vi "DrawPathAndRobotOnThatPath.vi"(6 "CenterOfRotYOffset (px)":dbl=20.0, 7 "PathMode":enum16{"Left", "Right", "Center"}(ring)=enum."Center", 8 "RobotLength (px)":dbl=40.0, 9 "RobotWidth (px)":dbl=30.0, 10 "Path (px)":cluster{dbl, dbl}[](array[cluster]), 11 "Image In":T1) -> (2 "NewPath (px)":cluster{dbl, dbl}[](array[cluster]), 3 "Image Out":T1)   [LabVIEW 2020]
uses:
  <vilib>/vision/Image Controls.llb/IMAQ Image.ctl
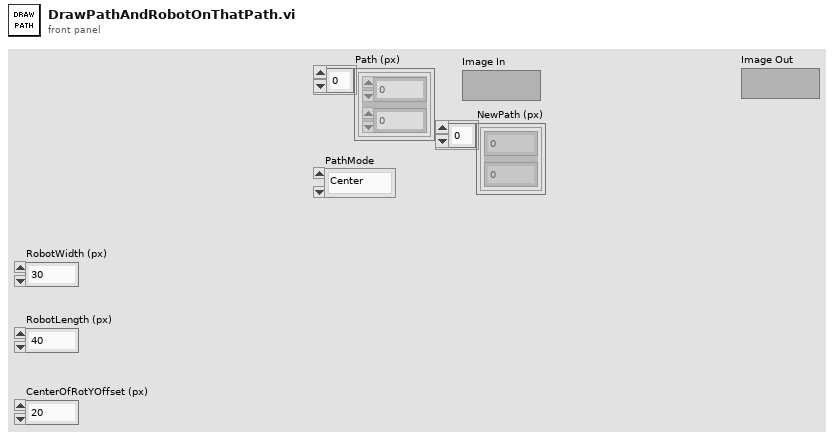
[diagram p1: front panel]
types:
  T1 = typedef "IMAQ Image.ctl" = refnum<image>
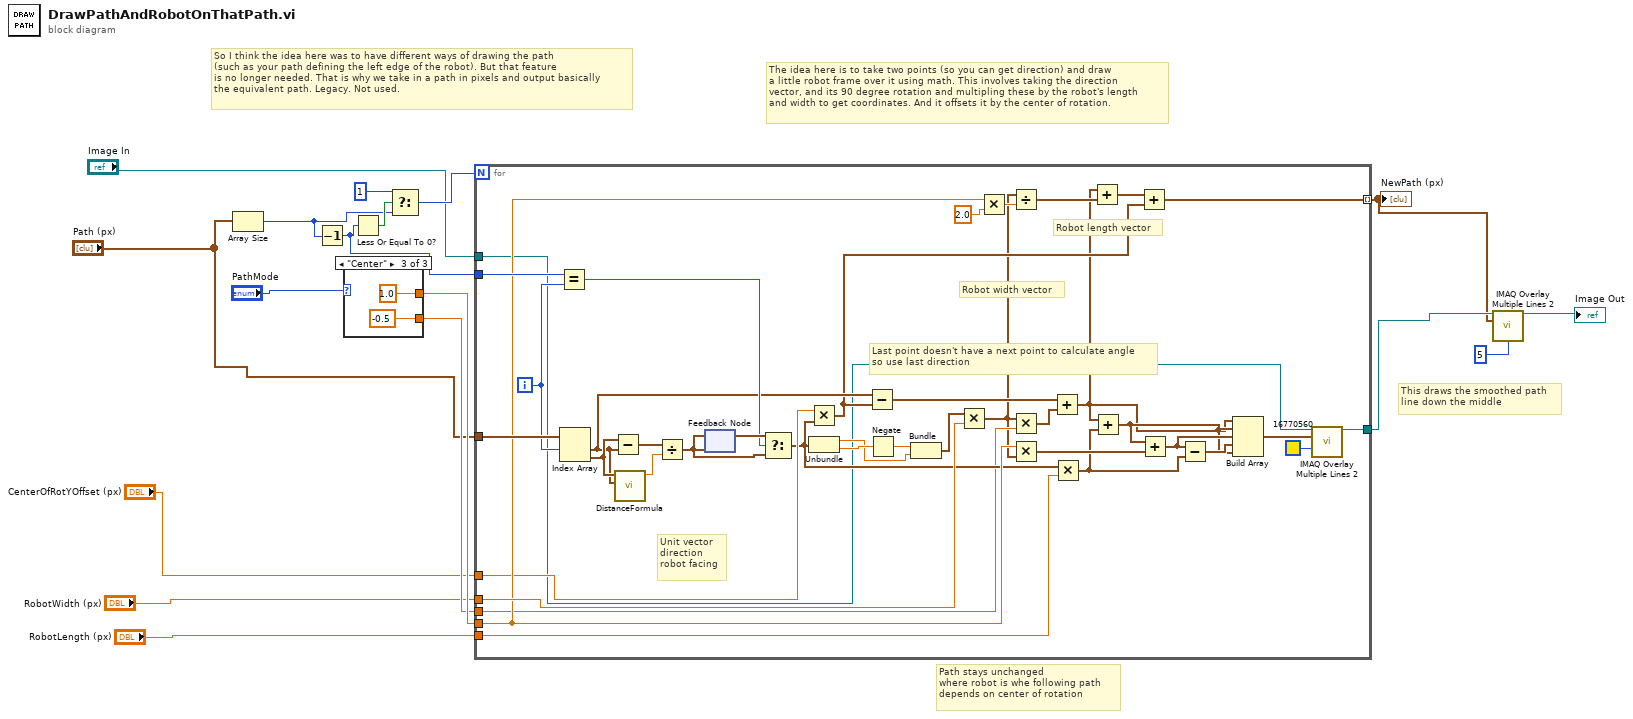
[diagram p0: block diagram]
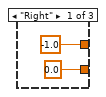
[diagram p2: hidden frame]
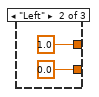
[diagram p3: hidden frame]
diagram:
  # "This draws the smoothed path\nline down the middle"
  # "The idea here is to take two points (so you can get direction) and draw\na little robot frame over it using math. This involves taking the direction\nvector, and its 90 degree rotation and multipling these by the robot's length\nand width to get coordinates. And it offsets it by the center of rotation."
  # "So I think the idea here was to have different ways of drawing the path\n(such as your path defining the left edge of the robot). But that feature\nis no longer needed. That is why we take in a path in pixels and output basically\nthe equivalent path. Legacy. Not used."
  # "Path stays unchanged\nwhere robot is whe following path\ndepends on center of rotation"
  n1 = Array Size(array="Path (px)") -> (size(s)=w14:i32)
  n2 = Decrement(x=w14) -> (x-1=w13:i32)
  n3 = case shown="\"Center\"" "PathMode" {
    tunnel: [-1.0 ("y") 1.0 ("y") 1.0 ("y")] -> w12
    tunnel: [0.0 ("y") 0.0 ("y") -0.5 ("y")] -> w11
    frame "Right" {
    }
    frame "Left" {
    }
    frame "Center" {
    }
  }
  n4 = Less Or Equal To 0?(x=w13) -> (x <= 0?=w17:bool)
  n5 = Select(t=1 ("y"), s=w17, f=w14) -> (s? t:f=w15:i32)
  n6 = for {
    N: w15 -> [_]
    tunnel: "Image In" -> [w25]
    tunnel: [w62] -> w2
    tunnel: "Path (px)" -> [w61]
    tunnel: w12 -> [w40]
    tunnel: "RobotLength (px)" -> [w59]
    tunnel: "RobotWidth (px)" -> [w58]
    tunnel: w13 -> [w45]
    tunnel: [w32] -> w1 mode=indexing
    tunnel: "CenterOfRotYOffset (px)" -> [w38]
    tunnel: w11 -> [w28]
    i -> [w46]
    # "Last point doesn't have a next point to calculate angle\nso use last direction"
    # "Robot width vector"
    # "Robot length vector"
    # "Unit vector\ndirection\nrobot facing"
    n7 = Equal?(x=w45, y=w46) -> (x = y?=w43:bool)
    n8 = Index Array(array=w61, index #1=w46) -> (element #1=w34:cluster{dbl, dbl}, element #2=w60:cluster{dbl, dbl})  [unwired: 1 in]
    n9 = Subtract(x=w60, y=w34) -> (x-y=w55:cluster{dbl, dbl})
    n10 = call "DistanceFormula.vi"("Point 2"=w34, "Point 1"=w60) -> ("Distance"=w54:dbl)  [unwired: 9 in]
    n11 = Divide(x=w55, y=w54) -> (x/y=w36:cluster{dbl, dbl})
    n12 = feedback-in #1(w36) -> ()
    n13 = feedback #1(w36) -> (w44:cluster{dbl, dbl})
    n14 = Select(t=w44, s=w43, f=w36) -> (s? t:f=w31:cluster{dbl, dbl})
    n15 = Multiply(x=w38, y=w31) -> (x*y=w33:cluster{dbl, dbl})
    n16 = Unbundle(w31) -> (w47:dbl, w53:dbl)
    n17 = Subtract(x=w34, y=w33) -> (x-y=w30:cluster{dbl, dbl})
    n18 = Negate(x=w53) -> (-x=w52:dbl)
    n19 = Bundle(w52, w47) -> (w51:cluster{dbl, dbl})  [unwired: 1 in]
    n20 = Multiply(x=w51, y=w58) -> (x*y=w27:cluster{dbl, dbl})
    n21 = Multiply(x=w40, y=2.0) -> (x*y=w39:dbl)
    n22 = Divide(x=w27, y=w39) -> (x/y=w42:cluster{dbl, dbl})
    n23 = Multiply(x=w27, y=w28) -> (x*y=w29:cluster{dbl, dbl})
    n24 = Multiply(x=w40, y=w27) -> (x*y=w41:cluster{dbl, dbl})
    n25 = Add(x=w30, y=w29) -> (x+y=w26:cluster{dbl, dbl})
    n26 = Multiply(x=w31, y=w59) -> (x*y=w37:cluster{dbl, dbl})
    n27 = Add(x=w26, y=w42) -> (x+y=w35:cluster{dbl, dbl})
    n28 = Add(x=w26, y=w37) -> (x+y=w50:cluster{dbl, dbl})
    n29 = Add(x=w35, y=w33) -> (x+y=w32:cluster{dbl, dbl})
    n30 = Add(x=w50, y=w41) -> (x+y=w49:cluster{dbl, dbl})
    n31 = Subtract(x=w49, y=w37) -> (x-y=w48:cluster{dbl, dbl})
    n32 = Build Array(w26, w50, w49, w48, w26) -> (w56:cluster{dbl, dbl}[])
    n33 = call "IMAQ Overlay Multiple Lines 2"("Image"=w25, "Line End Points"=w56, "Color"=u32 16770560) -> ("Image Out"=w62:T1)  [unwired: 11 in, 1 out]
  }
  "NewPath (px)" <- w1
  n34 = call "IMAQ Overlay Multiple Lines 2"("Image"=w2, "Line End Points"=w1, "Width"=u32 5) -> ("Image Out"=→"Image Out":T1)  [unwired: 11 in, 1 out]
